vi "MultiDepth Physical Learning.vi"(0 "FPGA VI Reference In":refnum<k20>, 1 "Input RUY":T5, 2 "Change Depth?":bool, 5 "Prev Posit Cluster":T4={"Prev L1 to L4 Posit"=[-0.5319, -0.035669172703475985, -2.0566170657346783, 0.9099264705882353], "Prev Stage Posit"=[6.002553885707208, 5.996566124542428, 5.995469940427586], "Prev OCT Z Posit"=-0.0}, 9 "Offset Home 2 RCM":dbl[](array[numeric])=[0.0, 0.0, 0.0, 0.0], 11 "error in":errorcluster, 12 "PID Cluster":T1={"L1 to L4 PID Cluster"={"L1 PID Gains"={"Kp"=0.005, "Kd"=0.5, "Ki"=0.0005}, "L2 PID Gains"={"Kp"=0.01, "Kd"=1.0, "Ki"=0.005}, "L3 PID Gains"={"Kp"=0.05, "Kd"=1.0, "Ki"=0.0005}, "L4 PID Gains"={"Kp"=0.1, "Kd"=0.1, "Ki"=0.0005}}, "Stage PID Cluster"={"Stage Z PID"={"Kp"=0.0005, "Kd"=0.001, "Ki"=0.0}, "Stage Y PID"={"Kp"=0.0003, "Kd"=0.01, "Ki"=0.0}, "Stage X PID"={"Kp"=0.0003, "Kd"=0.01, "Ki"=0.0}}, "OCT Z PID Gains"={"Kp"=0.0003, "Kd"=0.0001, "Ki"=0.01}}, 13 "Delta Ref":T2, 14 "Learning Gains":dbl[](array[numeric])=[1.0, 1.0, 1.0, 0.0]) -> (3 "Updated RUY":T5, 4 "FPGA VI Reference Out":refnum<k20>, 6 "Last Posit Cluster":T3={"Last L1 to L4 Posit"=[0.0, 0.0, 0.0, 0.0], "Last Stage Posit"=[6.0, 6.0, 6.0], "Last OCT Z Posit"=0.0}, 15 "error out":errorcluster)   [LabVIEW 2016]
uses:
  <vilib>/Platform/TimedLoop/XDataNode/timing_clust.ctl
  <vilib>/Platform/TimedLoop/XDataNode/nitl_modes.ctl
  <vilib>/Platform/TimedLoop/XDataNode/wakeup.ctl
  Global Variables.vi
  <vilib>/platform/TimedLoop/XDataNode/XDataNode.xnode
  <vilib>/Platform/TimedLoop/XDataNode/XDNodeRunTimeDep.lvlib
panel:
  out "In Servo Loop":bool
  out "Loading Finished":bool
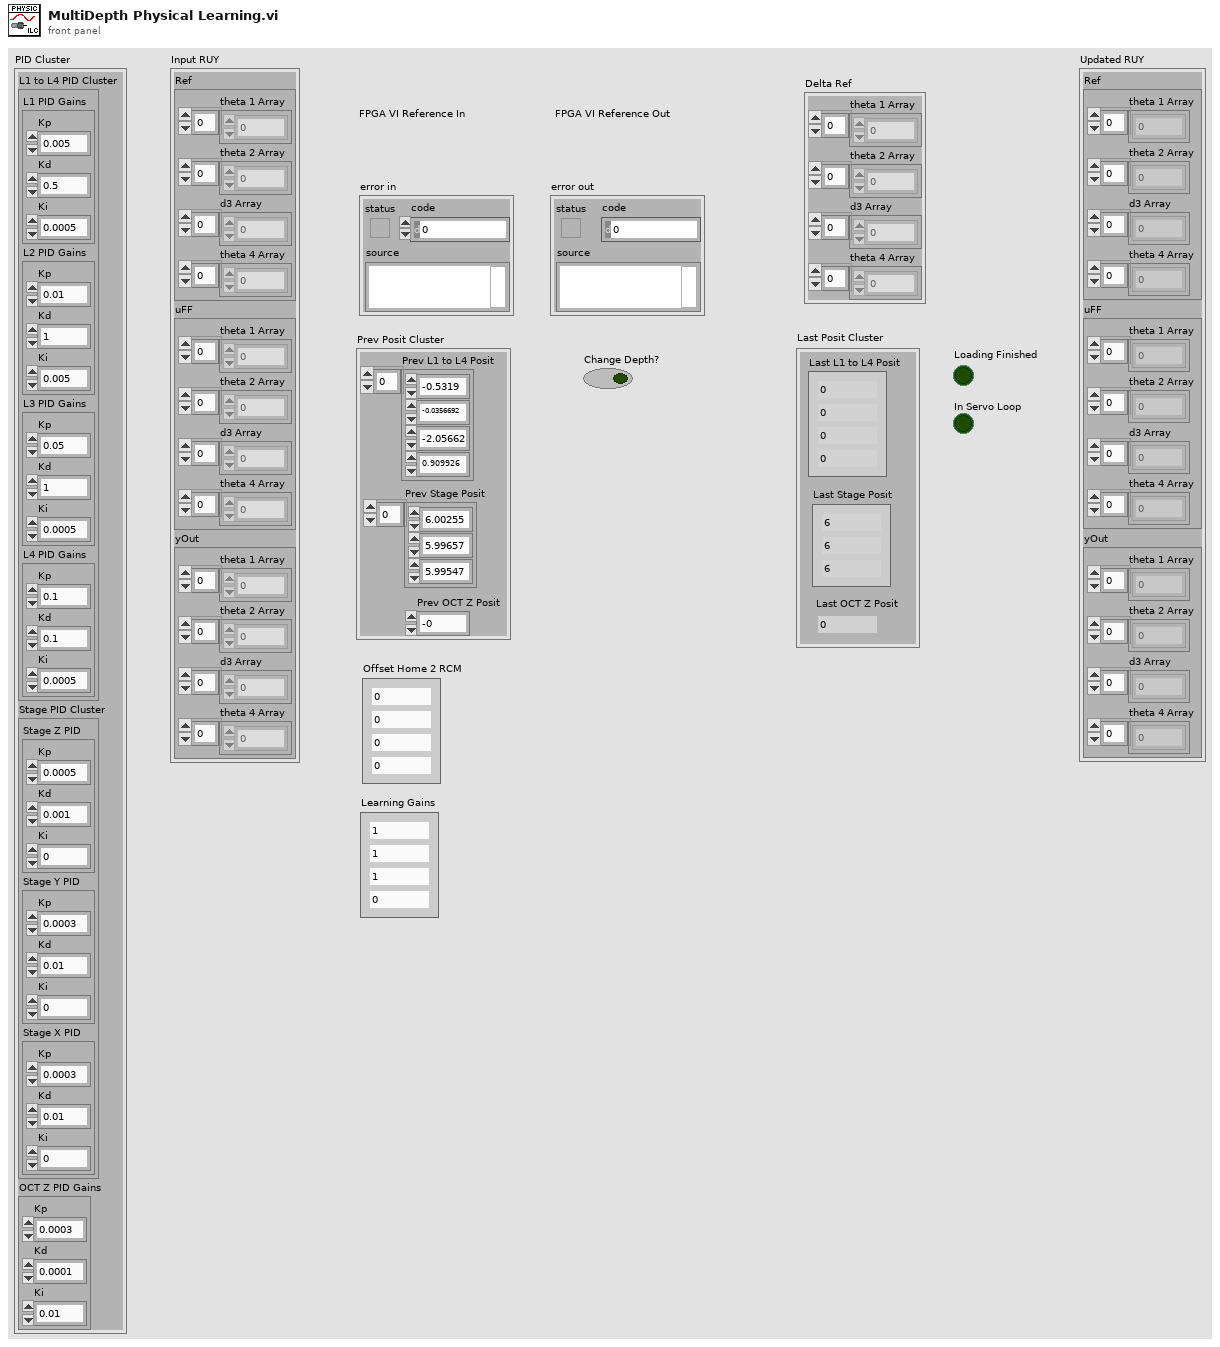
[diagram p1: front panel]
types:
  T1 = cluster{"L1 to L4 PID Cluster":cluster{"L1 PID Gains":cluster{"Kp":dbl, "Kd":dbl, "Ki":dbl}, "L2 PID Gains":cluster{"Kp":dbl, "Kd":dbl, "Ki":dbl}, "L3 PID Gains":cluster{"Kp":dbl, "Kd":dbl, "Ki":dbl}, "L4 PID Gains":cluster{"Kp":dbl, "Kd":dbl, "Ki":dbl}}, "Stage PID Cluster":cluster{"Stage Z PID":cluster{"Kp":dbl, "Kd":dbl, "Ki":dbl}, "Stage Y PID":cluster{"Kp":dbl, "Kd":dbl, "Ki":dbl}, "Stage X PID":cluster{"Kp":dbl, "Kd":dbl, "Ki":dbl}}, "OCT Z PID Gains":cluster{"Kp":dbl, "Kd":dbl, "Ki":dbl}}
  T2 = cluster{"theta 1 Array":dbl[], "theta 2 Array":dbl[], "d3 Array":dbl[], "theta 4 Array":dbl[]}
  T3 = cluster{"Last L1 to L4 Posit":dbl[], "Last Stage Posit":dbl[], "Last OCT Z Posit":dbl}
  T4 = cluster{"Prev L1 to L4 Posit":dbl[], "Prev Stage Posit":dbl[], "Prev OCT Z Posit":dbl}
  T5 = cluster{"Ref":cluster{"theta 1 Array":dbl[], "theta 2 Array":dbl[], "d3 Array":dbl[], "theta 4 Array":dbl[]}, "uFF":cluster{"theta 1 Array":dbl[], "theta 2 Array":dbl[], "d3 Array":dbl[], "theta 4 Array":dbl[]}, "yOut":cluster{"theta 1 Array":dbl[], "theta 2 Array":dbl[], "d3 Array":dbl[], "theta 4 Array":dbl[]}}
  T6 = cluster{"Stop Vacuum":bool, "Vacuum Force":i8, "Max Limit [mmHg]":dbl, "Slide in":i8, "Irrigation?":bool}
  T7 = typedef "XDNodeRunTimeDep.lvlib/timing_clust.ctl" = cluster{"Expected End [f-1]":u64, "Actual End [f-1]":u64, "Finished Late? [f-1]":bool, "Expected End [i-1]":u64, "Actual End [i-1]":u64, "Finished Late? [i-1]":bool, "Expected Start [i]":u64, "Actual Start [i]":u64, "Expected Start [f]":u64, "Actual Start [f]":u64, "Source Name":string, "Structure Name":string, "Period":i64, "Deadline":i64, "Offset":i64, "Start":i64, "Priority":i32, "Timeout":i32, "Mode":T8, "Wakeup Reason":T9, "Error":errorcluster, "Source Type":string, "Secondary Source Type":string, "Global End Time":u64, "Global Start Time":u64, "Frame Duration":u64, "Iteration Duration":u64, "Assigned CPU":i32, "I/O Scan Engine Mode":u32}
  T8 = typedef "XDNodeRunTimeDep.lvlib/nitl_modes.ctl" = enum32{"No Change", "Process missed periods, maintain original phase", "Discard missed periods, maintain original phase", "Process missed periods, ignore original phase", "Discard missed periods, ignore original phase"}
  T9 = typedef "XDNodeRunTimeDep.lvlib/wakeup.ctl" = enum32{"Normal", "Aborted", "Asynchronous wakeup", "Timing source error", "Timed loop error", "Timeout"}
  T10 = cluster{"L1 PID Gains":cluster{"Kp":dbl, "Kd":dbl, "Ki":dbl}, "L2 PID Gains":cluster{"Kp":dbl, "Kd":dbl, "Ki":dbl}, "L3 PID Gains":cluster{"Kp":dbl, "Kd":dbl, "Ki":dbl}, "L4 PID Gains":cluster{"Kp":dbl, "Kd":dbl, "Ki":dbl}}
  T11 = cluster{"Stage Z PID":cluster{"Kp":dbl, "Kd":dbl, "Ki":dbl}, "Stage Y PID":cluster{"Kp":dbl, "Kd":dbl, "Ki":dbl}, "Stage X PID":cluster{"Kp":dbl, "Kd":dbl, "Ki":dbl}}
  T12 = cluster{"Accurus button":bool[], "Accurus engaged?":bool, "Vacuum Force":i32, "Accurus Ch. A Vout":dbl, "Accurus Ch. B Vout":dbl, "Irrigation engaged?":bool}
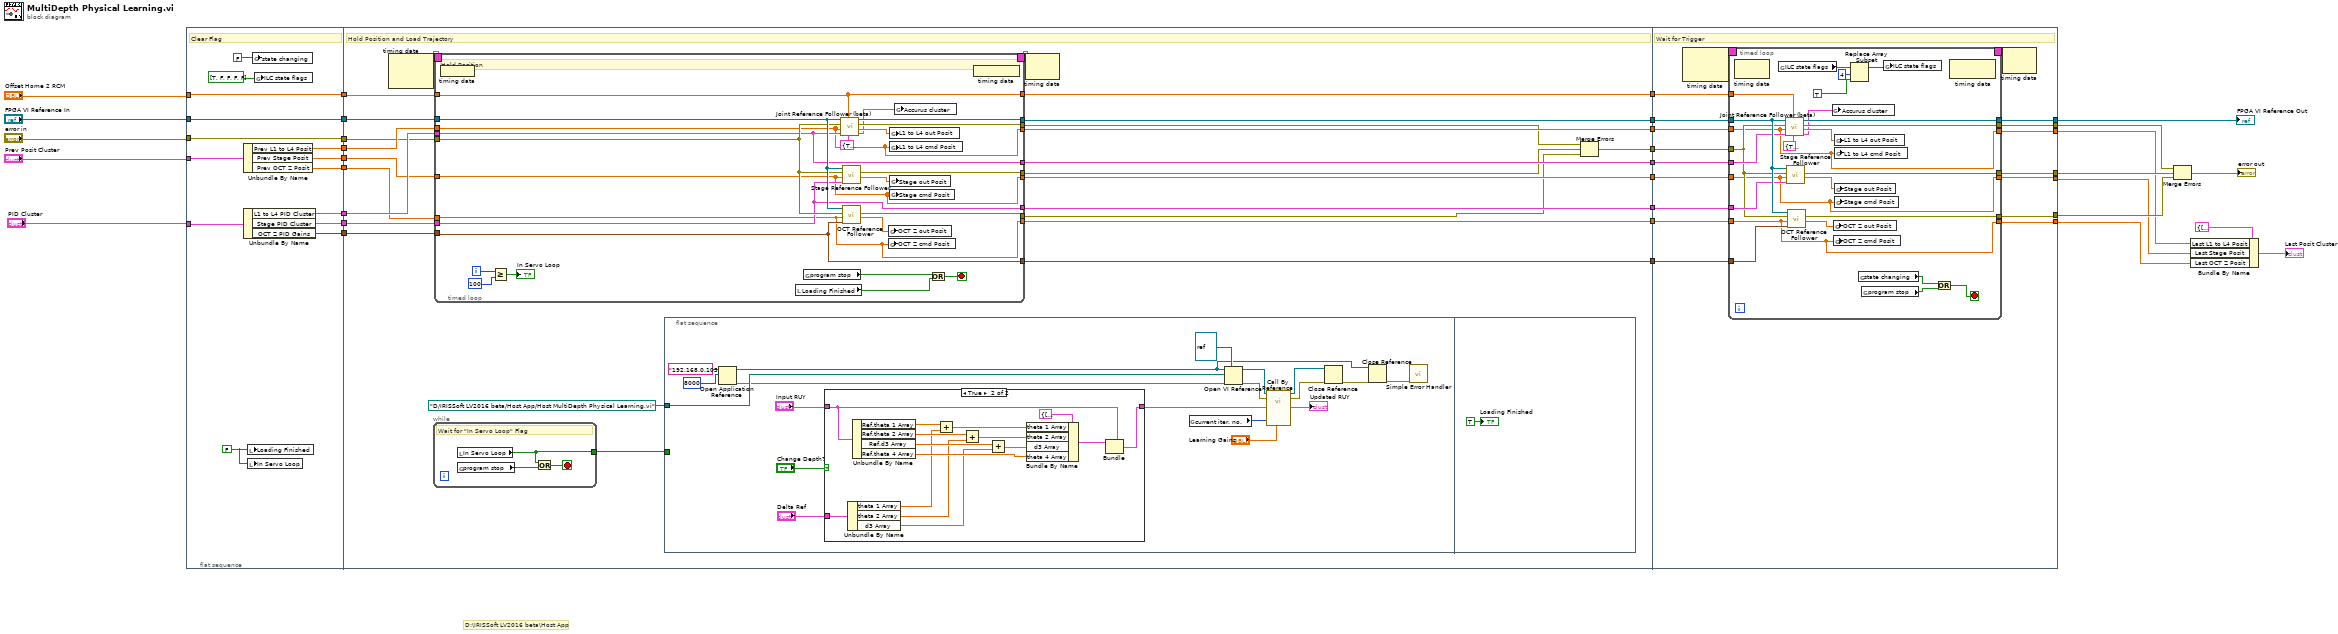
[diagram p0: block diagram]
diagram:
  # "D:\\IRISSoft LV2016 beta\\Host App"
  n1 = flat-sequence {
    tunnel: [w46] -> w33
    tunnel: "FPGA VI Reference In" -> [w46]
    tunnel: [w45] -> w32
    tunnel: "error in" -> [w45]
    tunnel: "Prev Posit Cluster" -> [w44]
    tunnel: "PID Cluster" -> [w43]
    tunnel: [w42] -> w31
    tunnel: [w41] -> w30
    tunnel: "Offset Home 2 RCM" -> [w40]
    tunnel: [w40] -> w29
    tunnel: [w39] -> w28
    tunnel: [w38] -> w27
    tunnel: [w37] -> w26
    tunnel: [w36] -> w25
    tunnel: w33 -> [w60]
    tunnel: w32 -> [w55]
    tunnel: w31 -> [w57]
    tunnel: w30 -> [w56]
    tunnel: w29 -> [w61]
    tunnel: w28 -> [w59]
    tunnel: w27 -> [w54]
    tunnel: w26 -> [w53]
    tunnel: w25 -> [w58]
    tunnel: [w72] -> w24
    tunnel: [w71] -> w23
    tunnel: [w70] -> w22
    tunnel: [w69] -> w21
    tunnel: [w68] -> w20
    tunnel: [w67] -> w19
    tunnel: [w66] -> w18
    tunnel: [w65] -> w17
    tunnel: [w49] -> w16
    tunnel: w24 -> [w155]
    tunnel: [w154] -> w9
    tunnel: [w153] -> w8
    tunnel: [w152] -> w7
    tunnel: w23 -> [w151]
    tunnel: w22 -> [w150]
    tunnel: w21 -> [w149]
    tunnel: w20 -> [w148]
    tunnel: w19 -> [w147]
    tunnel: w18 -> [w146]
    tunnel: w17 -> [w145]
    tunnel: [w144] -> w5
    tunnel: [w143] -> w4
    tunnel: [w142] -> w3
    tunnel: [w141] -> w1
    tunnel: w16 -> [w140]
    frame #0 {
      w35 = FALSE ("Loading Finished")
      # "Clear Flag"
      n2 = Unbundle By Name(w43) -> ("L1 to L4 PID Cluster"=w41:T10, "Stage PID Cluster"=w42:T11, "OCT Z PID Gains"=w36:cluster{"Kp":dbl, "Kd":dbl, "Ki":dbl})
      n3 = Unbundle By Name(w44) -> ("Prev L1 to L4 Posit"=w39:dbl[], "Prev Stage Posit"=w38:dbl[], "Prev OCT Z Posit"=w37:dbl)
      n4 = local write "Loading Finished"(w35) -> ()
      n5 = local write "In Servo Loop"(w35) -> ()
      n6 = global write "Global Variables.vi" "state changing"(FALSE ("state changing")) -> ()
      n7 = global write "Global Variables.vi" "ILC state flags"(bool[] [TRUE, FALSE, FALSE, FALSE, FALSE]) -> ()
    }
    frame #1 {
      # "Hold Position and Load Trajectory"
      n8 = node-c288() -> (w64:T7)  [unwired: 2 in]
      n9 = while {
        tunnel: [w74] -> w62
        stop <- w75 stop-if-true
        # "Wait for \"In Servo Loop\" Flag"
        n10 = local read "In Servo Loop"() -> (w74:bool)
        n11 = global read "Global Variables.vi" "program stop"() -> (w73:bool)
        n12 = Or(x=w74, y=w73) -> (x .or. y?=w75:bool)
      }
      n13 = timed-loop {
        timing: w64 -> [_]
        timing-out: [_] -> w63
        tunnel: w59 -> [w113]
        tunnel: w54 -> [w114]
        tunnel: w57 -> [w120]
        tunnel: w56 -> [w121]
        tunnel: w55 -> [w131]
        tunnel: w60 -> [w132]
        tunnel: w61 -> [w127]
        tunnel: w53 -> [w112]
        tunnel: w58 -> [w122]
        tunnel: [w113] -> w70
        tunnel: [w114] -> w69
        tunnel: [w112] -> w68
        tunnel: [w127] -> w71
        tunnel: [w126] -> w72
        tunnel: [w125] -> w52
        tunnel: [w124] -> w51
        tunnel: [w123] -> w50
        tunnel: [w122] -> w67
        tunnel: [w121] -> w66
        tunnel: [w120] -> w65
        i -> [w119]
        stop <- w135 stop-if-true
        # "Hold Position"
        n14 = node-c288 ("Output Node")() -> ()  [unwired: 1 in]
        n15 = Greater Or Equal?(x=w119, y=100) -> (x >= y?=→"In Servo Loop":bool)
        n16 = local read "Loading Finished"() -> (w134:bool)
        n17 = global read "Global Variables.vi" "program stop"() -> (w133:bool)
        n18 = call "Joint Reference Follower (beta).vi"("Accurus Ctrl Cluster"=T6 {"Stop Vacuum"=TRUE, "Vacuum Force"=0, "Max Limit [mmHg]"=600.0, "Slide in"=0, "Irrigation?"=TRUE}, "Offset Home2RCM [deg/mm]"=w127, "PID Ctrl Cluster"=w121, "Ref Array [deg/mm]"=w113, "error in"=w131, "FPGA VI Reference In"=w132) -> ("Accurus Output Cluster"=w115:T12, "Output Posit Array [deg/mm]"=w130:dbl[], "error out"=w125:errorcluster, "FPGA VI Reference Out"=w126:refnum<k20>)  [unwired: 2 in]
        n19 = call "Stage Reference Follower.vi"("Stage PID Cluster"=w120, "Stage cmd Posit [mm]"=w114, "error in"=w131, "FPGA VI Reference In"=w132) -> ("Stage out Posit [mm]"=w129:dbl[], "error out"=w124:errorcluster)  [unwired: 5 in, 1 out]
        n20 = call "OCT Reference Follower.vi"("OCT Z PID Gains"=w122, "OCT  Z cmd Posit [mm]"=w112, "error in"=w131, "FPGA VI Reference In"=w132) -> ("OCT  Z out Posit [mm]"=w128:dbl, "error out"=w123:errorcluster)  [unwired: 5 in, 1 out]
        n21 = global write "Global Variables.vi" "OCT Z out Posit"(w128) -> ()
        n22 = global write "Global Variables.vi" "OCT Z cmd Posit"(w112) -> ()
        n23 = global write "Global Variables.vi" "L1 to L4 out Posit"(w130) -> ()
        n24 = global write "Global Variables.vi" "L1 to L4 cmd Posit"(w113) -> ()
        n25 = global write "Global Variables.vi" "Stage out Posit"(w129) -> ()
        n26 = global write "Global Variables.vi" "Stage cmd Posit"(w114) -> ()
        n27 = global write "Global Variables.vi" "Accurus cluster"(w115) -> ()
        n28 = Or(x=w133, y=w134) -> (x .or. y?=w135:bool)
        n29 = node-c288() -> ()  [unwired: 1 out]
      }
      n30 = flat-sequence {
        tunnel: w62 -> [_]
        tunnel: path "D:/IRISSoft LV2016 beta/Host App/Host MultiDepth Physical Learning.vi" ("vi path") -> [w87]
        frame #0 {
          n31 = Open Application Reference(10:u16 8000 ("port number or service name (3363)"), 11:"192.168.0.105" ("machine name (\"\":  open local reference)")) -> (0:w84:errorcluster, 3:w89:refnum<vi>)  [unwired: 2 in]
          n32 = case shown="True" "Change Depth?" {
            tunnel: "Input RUY" -> [w95 w110]
            tunnel: [w95 w97] -> w78
            tunnel: "Delta Ref" -> [_ w108]
            frame False {
            }
            frame True {
              n33 = Unbundle By Name(w108) -> ("theta 1 Array"=w99:dbl[], "theta 2 Array"=w100:dbl[], "d3 Array"=w101:dbl[])
              n34 = Unbundle By Name(w110) -> ("Ref.theta 1 Array"=w109:dbl[], "Ref.theta 2 Array"=w106:dbl[], "Ref.d3 Array"=w104:dbl[], "Ref.theta 4 Array"=w102:dbl[])
              n35 = Add(x=w109, y=w99) -> (x+y=w107:dbl[])
              n36 = Add(x=w106, y=w100) -> (x+y=w105:dbl[])
              n37 = Add(x=w104, y=w101) -> (x+y=w103:dbl[])
              n38 = Bundle By Name(cluster=T2 {"theta 1 Array"=[], "theta 2 Array"=[], "d3 Array"=[], "theta 4 Array"=[]} ("Ref"), "theta 1 Array"=w107, "theta 2 Array"=w105, "d3 Array"=w103, "theta 4 Array"=w102) -> (w98:T2)
              n39 = Bundle(cluster=w110, "Ref"=w98) -> (w97:T5)  [unwired: 2 in]
            }
          }
          n40 = global read "Global Variables.vi" "current iter. no."() -> (w81:u16)
          n41 = Open VI Reference(type specifier VI Refnum (for type only)=refnum<vi> refnum, application reference (local)=w89, vi path=w87, error in (no error)=w84) -> (vi reference=w90:refnum<vi>, error out=w86:errorcluster)  [unwired: 2 in]
          n42 = call-by-ref "?"(reference=w90, error in=w86, "Learning Gains"="Learning Gains", "Curr Iter No"=w81, "Input RUY"=w78) -> (reference out=w91:refnum<vi>, error out=w85:errorcluster, "Updated RUY"=→"Updated RUY":T5)  [unwired: 8 in]
          n43 = Close Reference(reference=w91, error in (no error)=w85) -> (error out=w88:errorcluster)
          n44 = Close Reference(reference=w89, error in (no error)=w88) -> (error out=w83:errorcluster)
          n45 = call <vilib>:"Simple Error Handler.vi"("error in (no error)"=w83) -> ()  [unwired: 4 in, 5 out]
        }
        frame #1 {
          "Loading Finished" <- TRUE ("Loading Finished")
        }
      }
      n46 = node-c288(w63) -> ()  [unwired: 1 out]
      n47 = Merge Errors(w52, w51, w50) -> (w49:errorcluster)
    }
    frame #2 {
      # "Wait for Trigger"
      n48 = node-c288() -> (w157:T7)  [unwired: 2 in]
      n49 = timed-loop {
        timing: w157 -> [_]
        timing-out: [_] -> w156
        tunnel: w155 -> [w175]
        tunnel: [w174] -> w153
        tunnel: [w173] -> w154
        tunnel: [w172] -> w152
        tunnel: w151 -> [w171]
        tunnel: w150 -> [w160]
        tunnel: w149 -> [w159]
        tunnel: w148 -> [w158]
        tunnel: w147 -> [w170]
        tunnel: w146 -> [w169]
        tunnel: w145 -> [w168]
        tunnel: [w160] -> w144
        tunnel: [w159] -> w143
        tunnel: [w158] -> w142
        tunnel: [w164] -> w141
        tunnel: w140 -> [w163]
        stop <- w182 stop-if-true
        n50 = node-c288() -> ()  [unwired: 1 in, 1 out]
        n51 = global read "Global Variables.vi" "ILC state flags"() -> (w179:bool[])
        n52 = call "Joint Reference Follower (beta).vi"("Accurus Ctrl Cluster"=T6 {"Stop Vacuum"=TRUE, "Vacuum Force"=0, "Max Limit [mmHg]"=600.0, "Slide in"=0, "Irrigation?"=TRUE}, "Offset Home2RCM [deg/mm]"=w171, "PID Ctrl Cluster"=w169, "Ref Array [deg/mm]"=w160, "error in"=w163, "FPGA VI Reference In"=w175) -> ("Accurus Output Cluster"=w161:T12, "Output Posit Array [deg/mm]"=w167:dbl[], "error out"=w174:errorcluster, "FPGA VI Reference Out"=w164:refnum<k20>)  [unwired: 2 in]
        n53 = call "Stage Reference Follower.vi"("Stage PID Cluster"=w168, "Stage cmd Posit [mm]"=w159, "error in"=w163, "FPGA VI Reference In"=w175) -> ("Stage out Posit [mm]"=w166:dbl[], "error out"=w173:errorcluster)  [unwired: 5 in, 1 out]
        n54 = call "OCT Reference Follower.vi"("OCT Z PID Gains"=w170, "OCT  Z cmd Posit [mm]"=w158, "error in"=w163, "FPGA VI Reference In"=w175) -> ("OCT  Z out Posit [mm]"=w165:dbl, "error out"=w172:errorcluster)  [unwired: 5 in, 1 out]
        n55 = global write "Global Variables.vi" "Accurus cluster"(w161) -> ()
        n56 = global write "Global Variables.vi" "OCT Z out Posit"(w165) -> ()
        n57 = global write "Global Variables.vi" "OCT Z cmd Posit"(w158) -> ()
        n58 = global write "Global Variables.vi" "L1 to L4 out Posit"(w167) -> ()
        n59 = global write "Global Variables.vi" "L1 to L4 cmd Posit"(w160) -> ()
        n60 = global write "Global Variables.vi" "Stage out Posit"(w166) -> ()
        n61 = global write "Global Variables.vi" "Stage cmd Posit"(w159) -> ()
        n62 = Replace Array Subset(array=w179, new element=TRUE ("new element/subarray"), index=4) -> (w178:bool[])
        n63 = global read "Global Variables.vi" "state changing"() -> (w181:bool)
        n64 = global read "Global Variables.vi" "program stop"() -> (w180:bool)
        n65 = global write "Global Variables.vi" "ILC state flags"(w178) -> ()
        n66 = Or(x=w181, y=w180) -> (x .or. y?=w182:bool)
        n67 = node-c288() -> ()  [unwired: 1 in, 1 out]
      }
      n68 = node-c288(w156) -> ()  [unwired: 1 out]
    }
  }
  n69 = Merge Errors(w8, w9, w7) -> (→"error out":errorcluster)
  n70 = Bundle By Name(cluster=T3 {"Last L1 to L4 Posit"=[0.0, 0.0, 0.0, 0.0], "Last Stage Posit"=[6.0, 6.0, 6.0], "Last OCT Z Posit"=0.0} ("Last Posit Cluster 2"), "Last L1 to L4 Posit"=w5, "Last Stage Posit"=w4, "Last OCT Z Posit"=w3) -> (→"Last Posit Cluster":T3)
  "FPGA VI Reference Out" <- w1
